vi "Arduino Network Device Scan.vi"(2 "Resource index":i32) -> (0 "Network device table":string[][](table))   [LabVIEW 2020]
uses:
  Instrument drivers/Arduino/ctls_and_globals/Arduino tx msg cluster.ctl
  Instrument drivers/Arduino/ctls_and_globals/Arduino Global.vi
panel:
  in  "End addr.":u8=255
  in  "Start addr.":u8=1 min=1
  out "Current address":u8(slide) scale=0.0..255.0
  # "PN 12/06/2014"
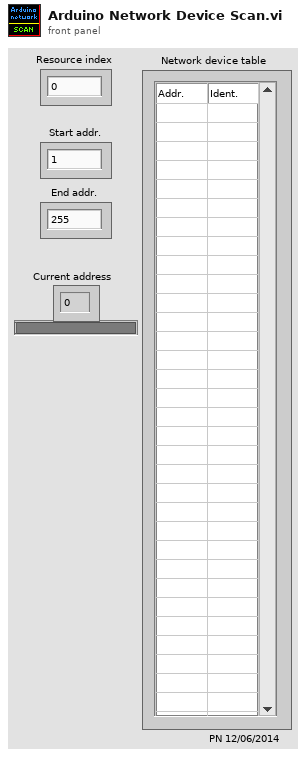
[diagram p1: front panel]
types:
  T1 = typedef "Arduino Config & resource typedef.ctl" = cluster{"baud rate (bps)":u32, "timeout (ms)":u32, "data bits":u16, "parity":enum16{"None", "Odd", "Even", "Mark", "Space"}, "stop bits (10: 1 bit)":u16, "flow control":u16, "termination char (hex)":u8, "Enable Termination Char":bool, "byte count":u32, "Resource locked?":bool, "VISA resource name":refnum<visa-resource-name>}
  T2 = typedef "Arduino tx msg cluster.ctl" = cluster{"dest":u8, "A/D/C/I":string, "R/W":string, "chan":u8, "val (float)":sgl}
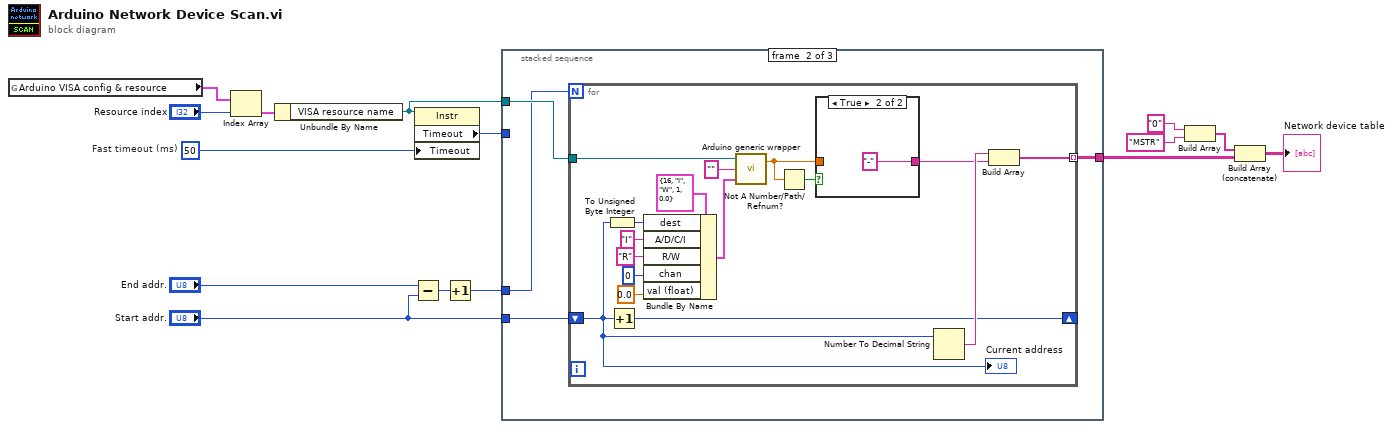
[diagram p0: block diagram]
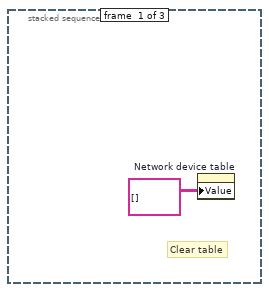
[diagram p2: hidden frame]
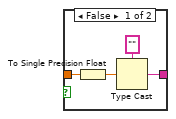
[diagram p3: hidden frame]
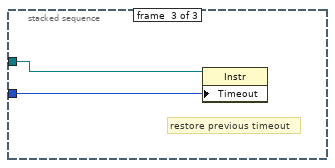
[diagram p4: hidden frame]
diagram:
  w15 = u32 50  # Fast timeout (ms)
  n1 = global read "Arduino Global.vi" "Arduino VISA config & resource"() -> (w11:T1[])
  n2 = Index Array(array=w11, index="Resource index") -> (element=w10:T1)
  n3 = Unbundle By Name(w10) -> ("VISA resource name"=w13:refnum<visa-resource-name>)
  n4 = Subtract(x="End addr.", y="Start addr.") -> (x-y=w2:u8)
  n5 = property class="Instr"(reference=w13, "Timeout"=w15) -> ("Timeout"=w14:u32)  [unwired: 1 in, 2 out]
  n6 = Increment(x=w2) -> (x+1=w1:u8)
  n7 = stacked-sequence {
    tunnel: w14 -> [_ _ w43]
    tunnel: w13 -> [_ w20 w42]
    tunnel: [_ w19 _] -> w6
    tunnel: "Start addr." -> [_ w18 _]
    tunnel: w1 -> [_ w17 _]
    frame #0 {
      # "Clear table"
      n8 = property on="Network device table" class="Tbl (strict)"("Value"=string[][] [] ("Network device table")) -> ()  [unwired: 2 in, 2 out]
    }
    frame #1 {
      n9 = for {
        N: w17 -> [_]
        tunnel: w20 -> [w29]
        tunnel: [w27] -> w19 mode=indexing
        shift-right: [w25] -> _
        shift-left: w18 -> [w26]
        n10 = To Unsigned Byte Integer(number=w26) -> (unsigned 8bit integer=w34:u8)
        n11 = Increment(x=w26) -> (x+1=w25:u8)
        n12 = Bundle By Name(cluster=T2 {"dest"=16, "A/D/C/I"="I", "R/W"="W", "chan"=1, "val (float)"=0.0} ("Tx msg cluster"), "dest"=w34, "A/D/C/I"="I" ("A/D/C"), "R/W"="R", "chan"=u8 0, "val (float)"=sgl 0.0) -> (w30:T2)
        n13 = call "Arduino generic wrapper.vi"("Tx msg cluster"=w30, "Channel Name"="", "Port name"=w29) -> ("Output"=w22:dbl)  [unwired: 1 out]
        n14 = Not A Number/Path/Refnum?(number/path/refnum=w22) -> (NaN/Path/Refnum?=w23:bool)
        n15 = case shown="True" w23 {
          tunnel: w22 -> [w38 _]
          tunnel: [w39 "-"] -> w21
          frame False {
            n16 = To Single Precision Float(number=w38) -> (single precision float=w37:sgl)
            n17 = Type Cast(type="", x=w37) -> (*(type *) &x=w39:string)
          }
          frame True {
          }
        }
        n18 = Number To Decimal String(number=w26) -> (decimal integer string=w28:string)  [unwired: 1 in]
        n19 = Build Array(w28, w21) -> (w27:string[])
        "Current address" <- w26
      }
    }
    frame #2 {
      # "restore previous timeout"
      n20 = property class="Instr"(reference=w42, "Timeout"=w43) -> ()  [unwired: 1 in, 2 out]
    }
  }
  n21 = Build Array("0", "MSTR") -> (w7:string[])
  n22 = Build Array (concatenate)(w7, w6) -> (→"Network device table":string[][])
